vi "HEIGHT_DIV_2.vi"() -> (0 "HEIGHT_DIV_2":i16=150)   [LabVIEW 2020]
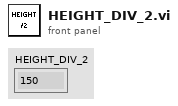
[diagram p1: front panel]
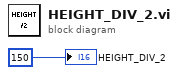
[diagram p0: block diagram]
diagram:
  "HEIGHT_DIV_2" <- i16 150
